vi "test 1.1.0 Mutation Adds Logging Section.vi"(8 "error in (no error)":errorcluster, 11 "TestCase in":refnum<class "Mutation.lvclass">) -> (0 "error out":errorcluster, 3 "TestCase out":refnum<class "Mutation.lvclass">)   [LabVIEW 2020, in "Mutation.lvclass"]
uses:
  Mutation.lvclass
  <vilib>/addons/_JKI Toolkits/VI Tester/TestCase.llb/TestCase.lvclass
  System Explorer/Implementation/Implementation.lvlib
  Scripting/AIM/AIM ARINC 429 Scripting.lvlib
  <vilib>/NI VeriStand/Custom Device Tools/Custom Device Utility Library/Custom Device Utility Library.lvlib
  C:/Program Files (x86)/National Instruments/LabVIEW 2020/vi.lib/addons/_JKI Toolkits/VI Tester/TestCase.llb/TestCase.lvclass
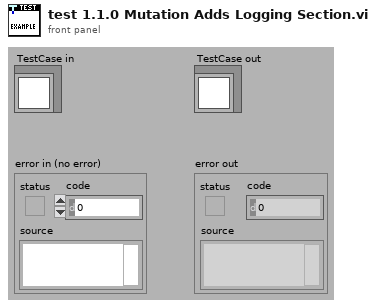
[diagram p1: front panel]
types:
  T1 = typedef "Custom Device API.lvlib/Custom Device Item Ref.ctl" = u64
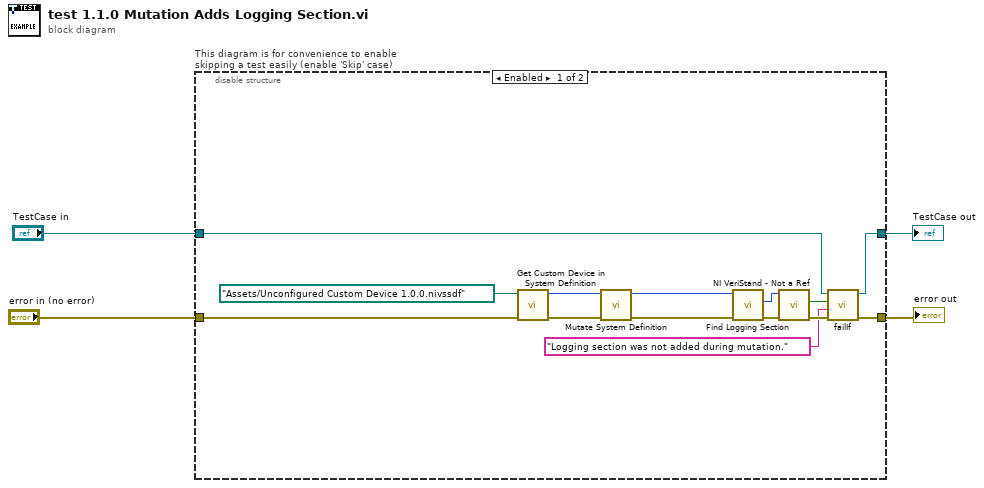
[diagram p0: block diagram]
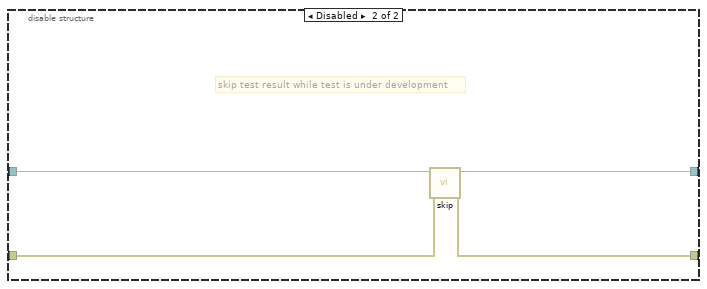
[diagram p2: hidden frame]
diagram:
  n1 = disable-structure "This diagram is for convenience to enable skipping a test easily (enable 'Skip' case)" shown="Enabled" {
    disable-tunnel: "TestCase in" -> [w8 w22]
    disable-tunnel: [w7 w20] -> w1
    disable-tunnel: [w9 w21] -> w3
    disable-tunnel: "error in (no error)" -> [w18 w19]
    frame Enabled {
      n2 = call "Get Custom Device in System Definition.vi"("error in (no error)"=w18, "system definition"=path "Assets/Unconfigured Custom Device 1.0.0.nivssdf" ("Absolute or Relative Path")) -> ("error out"=w16:errorcluster, "Ballard ARINC 429 custom device"=w15:u64)  [unwired: 8 in]
      n3 = call "Mutate System Definition.vi"("error in (no error)"=w16, "Device Ref in"=w15) -> ("error out"=w14:errorcluster, "Device Ref out"=w13:T1)  [unwired: 8 in]
      n4 = call "Find Logging Section.vi"("error in"=w14, "Ballard ARINC 429 custom device in"=w13) -> ("error out"=w11:errorcluster, "logging"=w12:T1)  [unwired: 7 in, 1 out]
      n5 = call <vilib>:"NI VeriStand - Not a Ref.vi"("error in (no error)"=w11, "Item Ref"=w12) -> ("error out"=w10:errorcluster, "Not a Ref"=w6:bool)  [unwired: 7 in, 1 out]
      n6 = call-dynamic "failIf.vi"("error in (no error)"=w10, "message (\"\")"="Logging section was not added during mutation." ("message (\"\")"), "fail"=w6, "TestCase in"=w8) -> ("error out"=w9:errorcluster, "TestCase out"=w7:refnum<class "Mutation.lvclass">)  [unwired: 6 in]
    }
    frame Disabled {
      # "skip test result while test is under development"
      n7 = call <vilib>:"skip.vi"("error in (no error)"=w19, "TestCase in"=w22) -> ("error out"=w21:errorcluster, "TestCase out"=w20:refnum<class "Mutation.lvclass">)  [unwired: 8 in]
    }
  }
  "error out" <- w3
  "TestCase out" <- w1
